vi "find.folders.with.dups.vi"() -> ()   [LabVIEW 2024]
panel:
  out "Numeric":i32
  out "currrent folder":string
  out "Array":path[](array[path])
  out "error out":errorcluster
  in  "Folder Path":path=path "D:/Comics/Marvel"
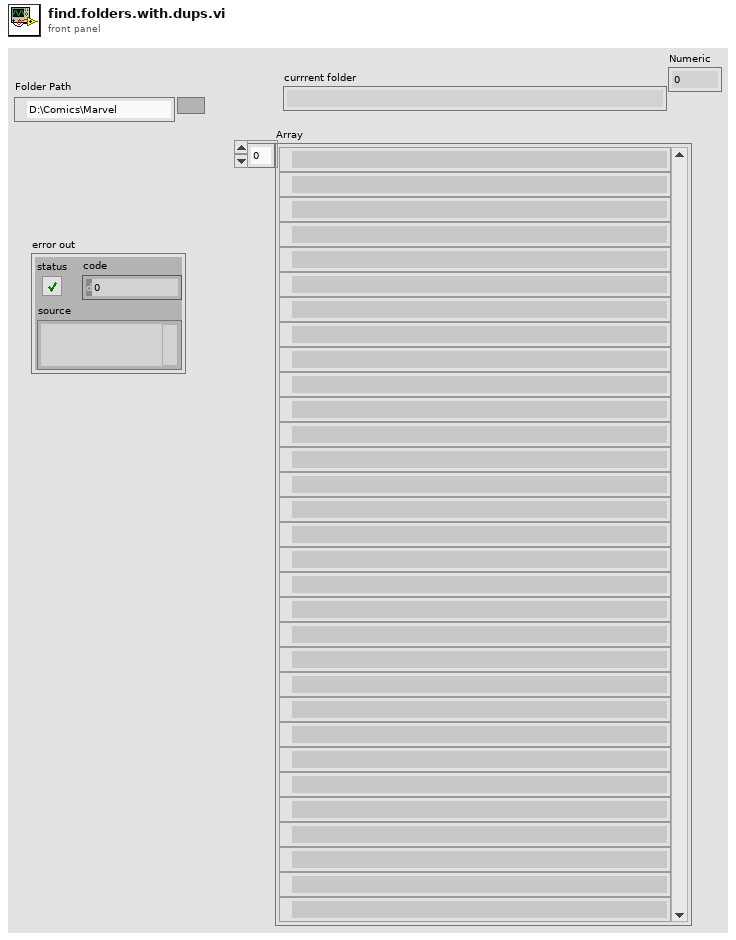
[diagram p1: front panel]
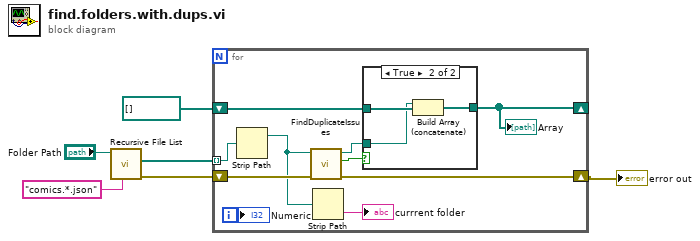
[diagram p0: block diagram]
diagram:
  n1 = call <vilib>:"Recursive File List.vi"("pattern"="comics.*.json", "Folder Path"="Folder Path") -> ("error out"=w3:errorcluster, "All Files in Dir"=w4:path[])  [unwired: 5 in, 3 out]
  n2 = for {
    tunnel: w4 -> [w16] mode=indexing
    shift-right: [w14] -> w2
    shift-left: w3 -> [w15]
    shift-right: [w10] -> _
    shift-left: path[] [] -> [w12]
    i -> [w7]
    n3 = Strip Path(path=w16) -> (stripped path=w9:path)  [unwired: 1 out]
    n4 = call "FindDuplicateIssues.vi"("error in"=w15, "path"=w9) -> ("error out"=w14:errorcluster, "dups found"=w13:bool, "path out"=w11:path)  [unwired: 7 in]
    n5 = Strip Path(path=w9) -> (name=→"currrent folder":string)  [unwired: 1 out]
    n6 = case shown="True" w13 {
      tunnel: w12 -> [w17 w20]
      tunnel: [w17 w19] -> w10
      tunnel: w11 -> [_ w18]
      frame False {
      }
      frame True {
        n7 = Build Array (concatenate)(w18, w20) -> (w19:path[])
      }
    }
    "Array" <- w10
    "Numeric" <- w7
  }
  "error out" <- w2
